vi "Find Number of Lines.vi"(7 "Line Terminator (\\n)":string="\n", 11 "String":string) -> (3 "Number of Lines":i32)   [LabVIEW 2020]
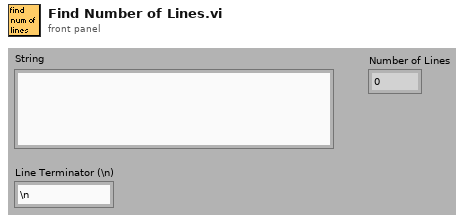
[diagram p1: front panel]
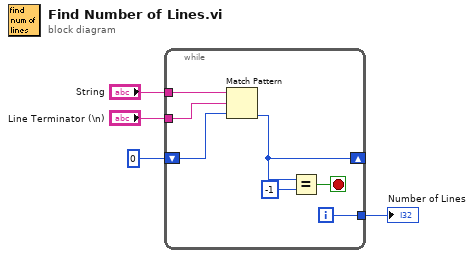
[diagram p0: block diagram]
diagram:
  n1 = while {
    tunnel: "String" -> [w10]
    shift-right: [w7] -> _
    shift-left: 0 ("offset past token") -> [w8]
    tunnel: "Line Terminator (\\n)" -> [w9]
    tunnel: [w11] -> w1
    i -> [w11]
    stop <- w5 stop-if-true
    n2 = Match Pattern(string=w10, regular expression=w9, offset (0)=w8) -> (offset past match=w7:i32)  [unwired: 3 out]
    n3 = Equal?(x=w7, y=-1) -> (x = y?=w5:bool)
  }
  "Number of Lines" <- w1
